vi "Text2Img.vi"(8 "error in (no error)":errorcluster, 11 "TextInfo":T2={"Text"="", "TextColor"={"Text BG"=0, "Text Color"=16448250}, "Size"=0, "FontDetails"={"Text.Font"={"Font Name"="Segoe UI", "Size"=29, "Bold"=FALSE, "Italic"=FALSE, "Underline"=FALSE, "Strikeout"=FALSE, "Color"=16448250}}}) -> (0 "error out":errorcluster, 3 "Image":T3(plugin-control))   [LabVIEW 2025]
uses:
  <vilib>/Utility/miscctls.llb/LVBoundsTypeDef.ctl
  <vilib>/vision/NI_Vision_Development_Module.lvlib
  Windows/Controls/Text2Img.ctl
panel:
  out "Stage1":string
  out "Stage2":string
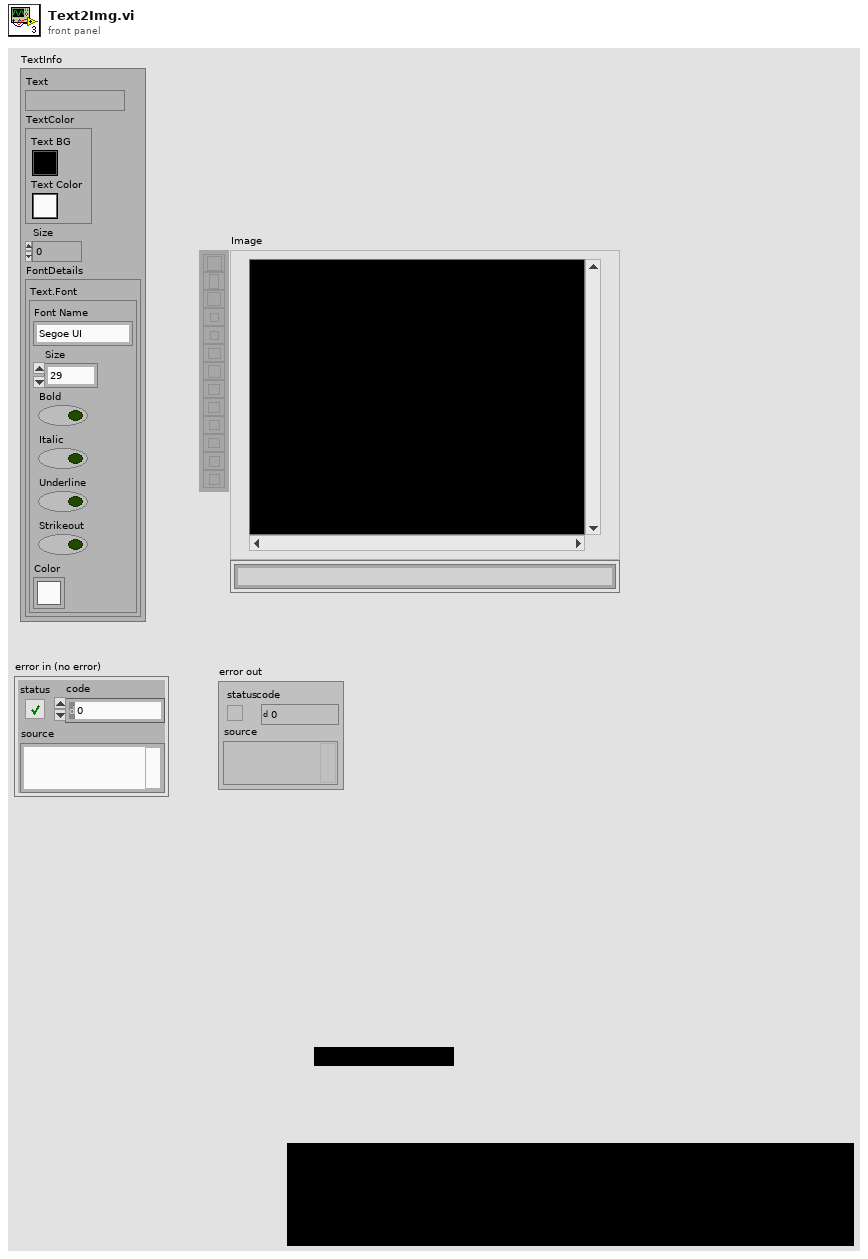
[diagram p1: front panel]
types:
  T1 = typedef "Text2Img.ctl" = cluster{"Text.Font":cluster{"Font Name":string, "Size":u16, "Bold":bool, "Italic":bool, "Underline":bool, "Strikeout":bool, "Color":u32}}
  T2 = cluster{"Text":string, "TextColor":cluster{"Text BG":u32, "Text Color":u32}, "Size":u16, "FontDetails":T1}
  T3 = typedef "IMAQ Image.ctl" = refnum<image>
  T4 = typedef "Image Type" = u32
  T5 = typedef "LVBoundsTypeDef.ctl" = cluster{"Width":u32, "Height":u32}
  T6 = cluster{"Font Name":string, "Size":u16, "Bold":bool, "Italic":bool, "Underline":bool, "Strikeout":bool, "Color":u32}
  T7 = typedef "imagedata.ctl" = cluster{"image type":i32, "image depth":i32, "image":u8[], "mask":u8[], "colors":u32[], "Rectangle":cluster{"left":i16, "top":i16, "right":i16, "bottom":i16}}
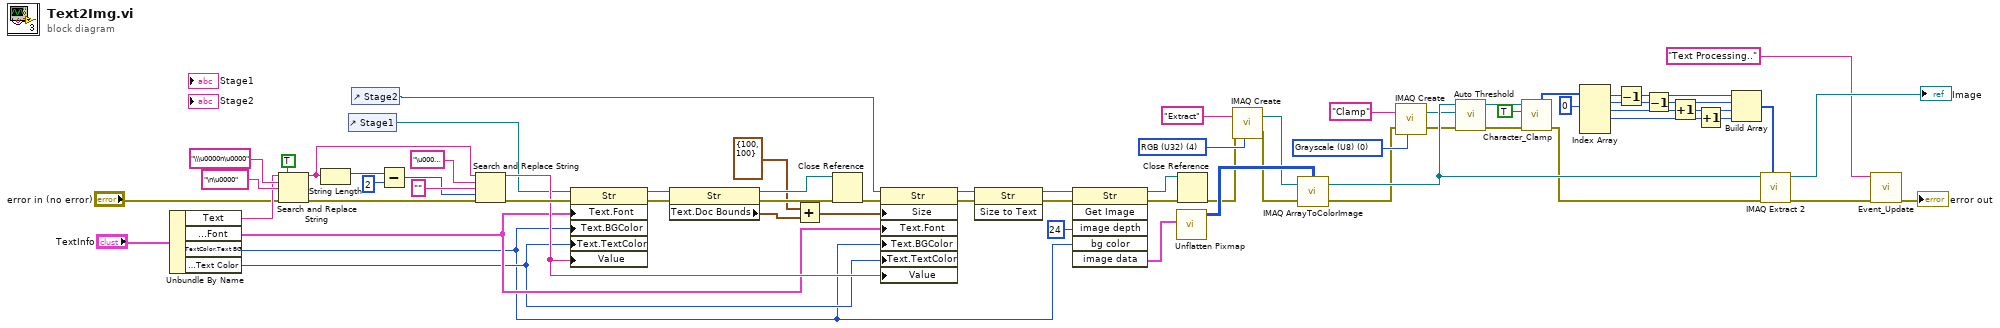
[diagram p0: block diagram]
diagram:
  w25 = T4 4 items=["Grayscale (U8)", "Grayscale (I16)", "Grayscale (SGL)", "Complex (CSG)", "RGB (U32)", "HSL (U32)", "RGB (U64)", "Grayscale (U16)"] ("Image Type")
  w45 = T4 0 items=["Grayscale (U8)", "Grayscale (I16)", "Grayscale (SGL)", "Complex (CSG)", "RGB (U32)", "HSL (U32)", "RGB (U64)", "Grayscale (U16)"] ("Image Type")
  n1 = Unbundle By Name("TextInfo") -> ("Text"=w9:string, "FontDetails.Text.Font"=w8:T6, "TextColor.Text BG"=w6:u32, "TextColor.Text Color"=w7:u32)
  n2 = Search and Replace String(replace all?=TRUE ("replace all? (F)"), input string=w9, search string="\\\u0000n\u0000" ("replace string (\"\")"), replace string="\n\u0000" ("replace string (\"\")"), error in="error in (no error)") -> (result string=w13:string, error out=w49:errorcluster)  [unwired: 3 in, 2 out]
  n3 = String Length(string=w13) -> (length=w53:i32)
  n4 = control-ref of="Stage1"() -> (w30:refnum<vi>)
  n5 = control-ref of="Stage2"() -> (w31:refnum<vi>)
  n6 = Subtract(x=w53, y=2) -> (x-y=w51:i32)
  n7 = Search and Replace String(input string=w13, search string="\u0000\u0000" ("replace string (\"\")"), replace string="" ("replace string (\"\")"), offset=w51, error in=w49) -> (result string=w47:string, error out=w48:errorcluster)  [unwired: 3 in, 2 out]
  n8 = property on="Property Node" class="Str"(reference=w30, error in=w48, "Text.Font"=w8, "Text.BGColor"=w6, "Text.TextColor"=w7, "Value"=w47) -> (reference out=w67:refnum<vi>, error out=w65:errorcluster)
  n9 = property on="Property Node" class="Str"(reference=w67, error in=w65) -> (reference out=w59:refnum<vi>, error out=w66:errorcluster, "Text.Doc Bounds"=w34:T5)
  n10 = Add(x=T5 {"Width"=100, "Height"=100}, y=w34) -> (x+y=w33:T5)
  n11 = Close Reference(reference=w59, error in (no error)=w66) -> (error out=w60:errorcluster)
  n12 = property on="Property Node" class="Str"(reference=w31, error in=w60, "Size"=w33, "Text.Font"=w8, "Text.BGColor"=w6, "Text.TextColor"=w7, "Value"=w47) -> (reference out=w27:refnum<vi>, error out=w29:errorcluster)
  n13 = invoke on="Invoke Node" class="Str" method="Size to Text"(reference=w27, error in=w29) -> (reference out=w26:refnum<vi>, error out=w28:errorcluster)  [unwired: 1 in, 1 out]
  n14 = invoke on="Invoke Node" class="Str" method="Get Image"(reference=w26, error in=w28, "image depth"=24 ("Image Depth"), "bg color"=w6) -> (reference out=w58:refnum<vi>, error out=w62:errorcluster, "image data"=w63:T7)  [unwired: 2 in, 3 out]
  n15 = call <vilib>:"Unflatten Pixmap.vi"("image data"=w63) -> ("24-bit pixmap"=w61:u32[][])  [unwired: 4 in, 6 out]
  n16 = Close Reference(reference=w58, error in (no error)=w62) -> (error out=w19:errorcluster)
  n17 = call "IMAQ Create"("Image Name"="Extract", "Image Type"=w25, "error in (no error)"=w19) -> ("New Image"=w24:T3, "error out"=w18:errorcluster)  [unwired: 2 in]
  n18 = call "IMAQ ArrayToColorImage"("Image Pixels (U32)"=w61, "Image"=w24, "error in (no error)"=w18) -> ("Image Out"=w21:T3, "error out"=w16:errorcluster)  [unwired: 2 in]
  n19 = call "IMAQ Create"("Image Name"="Clamp", "Image Type"=w45, "error in (no error)"=w16) -> ("New Image"=w15:T3, "error out"=w17:errorcluster)  [unwired: 2 in]
  n20 = call "Auto Threshold.vi"("Error In"=w17, "Grayscale Image"=w15, "RGB Image"=w21) -> ("Error Out"=w35:errorcluster, "Image Dst Out"=w20:T3)  [unwired: 5 in, 2 out]
  n21 = call "Character_Clamp.vi"("error in (no error)"=w35, "Measurement only"=TRUE, "U8 Character Image In"=w20) -> ("error out"=w14:errorcluster, "Clamp ROI"=w37:i32[])  [unwired: 6 in, 1 out]
  n22 = Index Array(array=w37, index #1=0 ("index")) -> (element #1=w41:i32, element #2=w40:i32, element #3=w43:i32, element #4=w42:i32)  [unwired: 3 in]
  n23 = Decrement(x=w41) -> (x-1=w39:i32)
  n24 = Decrement(x=w40) -> (x-1=w12:i32)
  n25 = Increment(x=w43) -> (x+1=w11:i32)
  n26 = Increment(x=w42) -> (x+1=w38:i32)
  n27 = Build Array(w39, w12, w11, w38) -> (w36:i32[])
  n28 = call "IMAQ Extract 2"("Optional Rectangle"=w36, "error in (no error)"=w14, "Image Src"=w21) -> ("error out"=w5:errorcluster, "Image Dst Out"=→"Image":T3)  [unwired: 7 in]
  n29 = call "Event_Update.vi"("Error In"=w5, "Event"="Text Processing..") -> ("Error Out"=→"error out":errorcluster)  [unwired: 9 in]
